vi "#125_MAV_MSG_POWER_STATUS_DECODE.vi"(11 "mavlink_payload":u8[](array[numeric])) -> (3 "POWER_STATUS":T1)   [LabVIEW 2023]
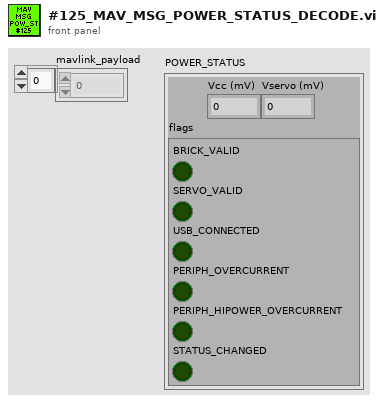
[diagram p1: front panel]
types:
  T1 = cluster{"Vcc (mV)":u16, "Vservo (mV)":u16, "flags":cluster{"BRICK_VALID":bool, "SERVO_VALID":bool, "USB_CONNECTED":bool, "PERIPH_OVERCURRENT":bool, "PERIPH_HIPOWER_OVERCURRENT":bool, "STATUS_CHANGED":bool}}
  T2 = cluster{"Vcc":u16, "Vservo":u16, "flags":cluster{"BRICK_VALID":bool, "SERVO_VALID":bool, "USB_CONNECTED":bool, "PERIPH_OVERCURRENT":bool, "PERIPH_HIPOWER_OVERCURRENT":bool, "STATUS_CHANGED":bool}}
  T3 = cluster{"Boolean array[0]":bool, "Boolean array[1]":bool, "Boolean array[2]":bool, "Boolean array[3]":bool, "Boolean array[4]":bool, "Boolean array[5]":bool}
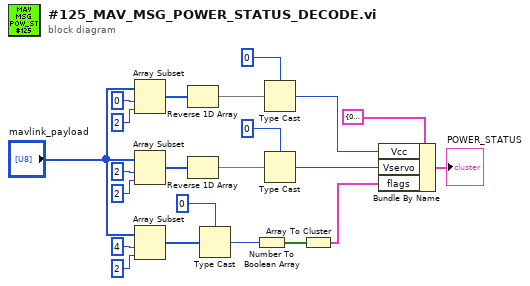
[diagram p0: block diagram]
diagram:
  n1 = Array Subset(array="mavlink_payload", index=0 ("Index"), length=2) -> (w19:u8[])
  n2 = Array Subset(array="mavlink_payload", index=2 ("Index"), length=2) -> (w13:u8[])
  n3 = Array Subset(array="mavlink_payload", index=4 ("Index"), length=2) -> (w3:u8[])
  n4 = Reverse 1D Array(array=w19) -> (reversed array=w18:u8[])
  n5 = Reverse 1D Array(array=w13) -> (reversed array=w12:u8[])
  n6 = Type Cast(type=u8 0 ("Index"), x=w3) -> (*(type *) &x=w4:u8)
  n7 = Number To Boolean Array(number=w4) -> (Boolean array=w1:bool[])
  n8 = Type Cast(type=u16 0 ("Index"), x=w18) -> (*(type *) &x=w15:u16)
  n9 = Type Cast(type=u16 0 ("Index"), x=w12) -> (*(type *) &x=w9:u16)
  n10 = Array To Cluster(array=w1) -> (cluster=w2:T3)
  n11 = Bundle By Name(cluster=T2 {"Vcc"=0, "Vservo"=0, "flags"={"BRICK_VALID"=FALSE, "SERVO_VALID"=FALSE, "USB_CONNECTED"=FALSE, "PERIPH_OVERCURRENT"=FALSE, "PERIPH_HIPOWER_OVERCURRENT"=FALSE, "STATUS_CHANGED"=FALSE}} ("POWER_STATUS"), "Vcc"=w15, "Vservo"=w9, "flags"=w2) -> (→"POWER_STATUS":T2)
